vi "Configure Bus Source (SPI-Clock).vi"(6 "Shift Direction (1: MSB)":i32(ring)=1 items=["LSB", "MSB"], 7 "Clock Source (10:Digital Channel 2)":u16(ring)=10 items=["Channel 1", "Channel 2", "Channel 3", "Channel 4", "Math 1", "Math 2", "Math 3", "Math 4", "Digital Channel 0", "Digital Channel 1", "Digital Channel 2", "Digital Channel 3", "Digital Channel 4", "Digital Channel 5", "Digital Channel 6", "Digital Channel 7", "Digital Channel 8", "Digital Channel 9", "Digital Channel 10", "Digital Channel 11", "Digital Channel 12", "Digital Channel 13", "Digital Channel 14", "Digital Channel 15"], 8 "error in (no error)":errorcluster, 9 "Polarity (0: Rise)":i32(ring) items=["Rise", "Fall"], 10 "BUS Number (0:Bus 1)":u8(ring) items=["Bus 1", "Bus 2", "Bus 3", "Bus 4", "Bus 5", "Bus 6", "Bus 7", "Bus 8", "Bus 9", "Bus 10", "Bus 11", "Bus 12", "Bus 13", "Bus 14", "Bus 15", "Bus 16"], 11 "VISA resource name":refnum<visa-resource-name>) -> (0 "error out":errorcluster, 3 "VISA resource name out":refnum<visa-resource-name>)   [LabVIEW 2015, in "Tektronix 7000 Series.lvlib"]
doc: "Configures SPI Bus Setting for an oscilloscope, only configures Clock relative part.\n\n<B>Note:</B> \nThese commands are not supported by TDS or CSA models."
uses:
  <instrlib>/Tektronix 7000 Series/Tektronix 7000 Series.lvlib
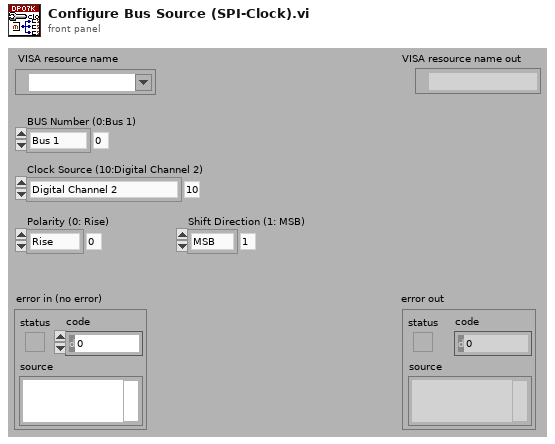
[diagram p1: front panel]
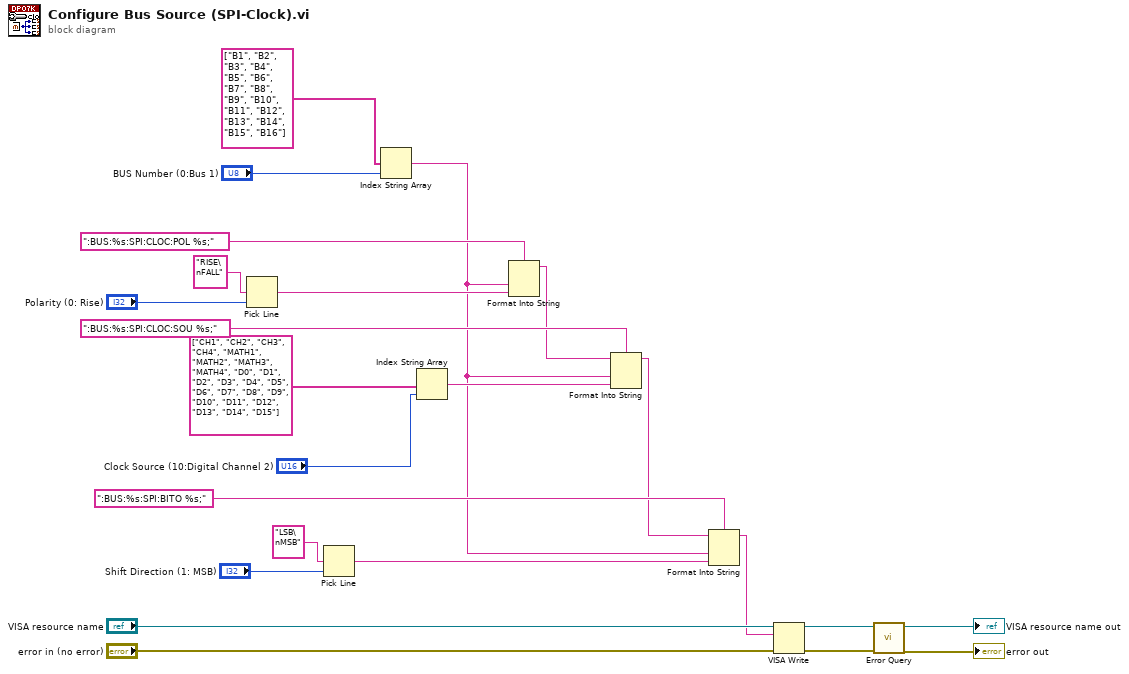
[diagram p0: block diagram]
diagram:
  n1 = Pick Line(multi-line string="RISE\nFALL", line index="Polarity (0: Rise)") -> (output string=w21:string)  [unwired: 1 out]
  n2 = Pick Line(multi-line string="LSB\nMSB", line index="Shift Direction (1: MSB)") -> (output string=w16:string)  [unwired: 1 out]
  n3 = Index String Array(1:"BUS Number (0:Bus 1)", 2:string[] ["B1", "B2", "B3", "B4", "B5", "B6", "B7", "B8", "B9", "B10", "B11", "B12", "B13", "B14", "B15", "B16"]) -> (0:w4:string)  [unwired: 1 out]
  n4 = Index String Array(1:"Clock Source (10:Digital Channel 2)", 2:string[] ["CH1", "CH2", "CH3", "CH4", "MATH1", "MATH2", "MATH3", "MATH4", "D0", "D1", "D2", "D3", "D4", "D5", "D6", "D7", "D8", "D9", "D10", "D11", "D12", "D13", "D14", "D15"]) -> (0:w7:string)  [unwired: 1 out]
  n5 = Format Into String(format string=":BUS:%s:SPI:CLOC:POL %s;", w4, w21) -> (resulting string=w6:string)  [unwired: 2 in, 1 out]
  n6 = Format Into String(format string=":BUS:%s:SPI:CLOC:SOU %s;", initial string=w6, w4, w7) -> (resulting string=w5:string)  [unwired: 1 in, 1 out]
  n7 = Format Into String(format string=":BUS:%s:SPI:BITO %s;", initial string=w5, w4, w16) -> (resulting string=w3:string)  [unwired: 1 in, 1 out]
  n8 = VISA Write(VISA resource name="VISA resource name", write buffer=w3, error in (no error)="error in (no error)") -> (VISA resource name out=w13:refnum<visa-resource-name>, error out=w12:errorcluster)  [unwired: 1 out]
  n9 = call <instrlib>:"Error Query.vi"("error in (no error)"=w12, "VISA resource name"=w13) -> ("error out"=→"error out":errorcluster, "VISA resource name out"=→"VISA resource name out":refnum<visa-resource-name>)  [unwired: 8 out]
